vi "Tabellen.vi"(8 "Fehler (Eingang, kein Fehler)":errorcluster) -> (0 "Fehler (Ausgang)":errorcluster, 1 "Tabelle Kontroll Interferent":string[][](array[string]), 2 "Tabbelle Referenz Interferent":string[][](array[string]), 3 "Tabelle Komponente":string[][](array[string]), 4 "Istwerte Komponente":string[](array[string]), 5 "Fehler Komponente":string[](array[string]), 7 "Max. Fehler Komponente":dbl)   [LabVIEW 2020, in "EPA 1065.lvlib" / "HovaCAL Interference verificaton.lvlib"]
uses:
  HovaCAL Interference verificaton.lvlib
  Aktion Index uebersetzten.ctl
  Linearisierung V2/Aktion Lin Daten aufarbeiten.ctl
  Linearisierung V2/Linearisierung v2.lvlib
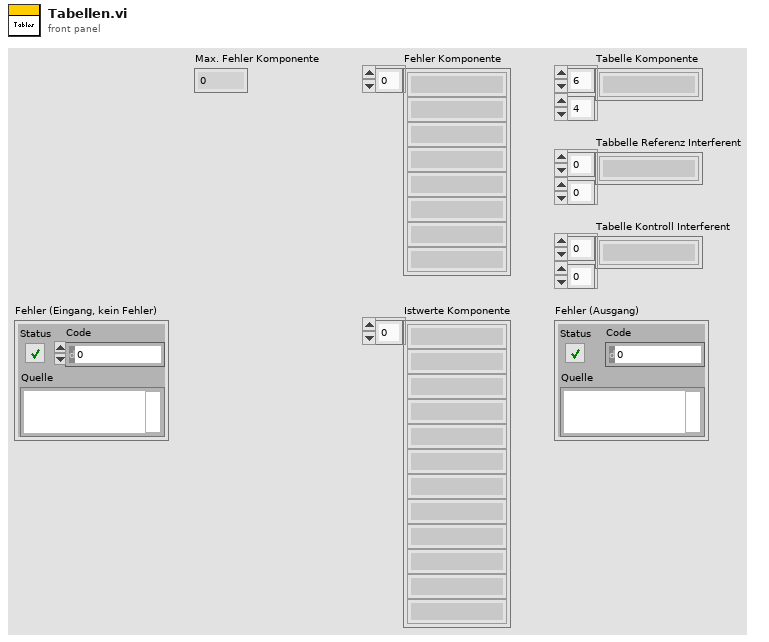
[diagram p1: front panel]
types:
  T1 = typedef "EPA 1065.lvlib/HovaCAL Interference verificaton.lvlib/Aktion Index uebersetzten.ctl" = enum16{"lesen", "schreiben", "auswerten", "Referenzwert", "KompIndex", "RefInterferIndex", "KontrInterfIndex"}
  T2 = typedef "Linearisierung v2.lvlib/Aktion Lin Daten aufarbeiten.ctl" = enum16{"lesen", "Protkolldaten", "speichern", "laden", "EPA auswerten", "Tabelle schreiben", "Lin auswerten", "Tab init", "Stufentabelle", "EPA aktiviert", "Nachbehandlung laden", "Tabelle löschen", "Istwerte löschen", "Zeile löschen", "Zeile einfügen", "LIN aktiviert", "LIN/EPA aktiv laden", "EGAK Tab", "LIN übernehmen", "Tab init ohne Stufen"}
  T3 = typedef "Linearisierung v2.lvlib/Eingabetabelle.ctl" = string[][]
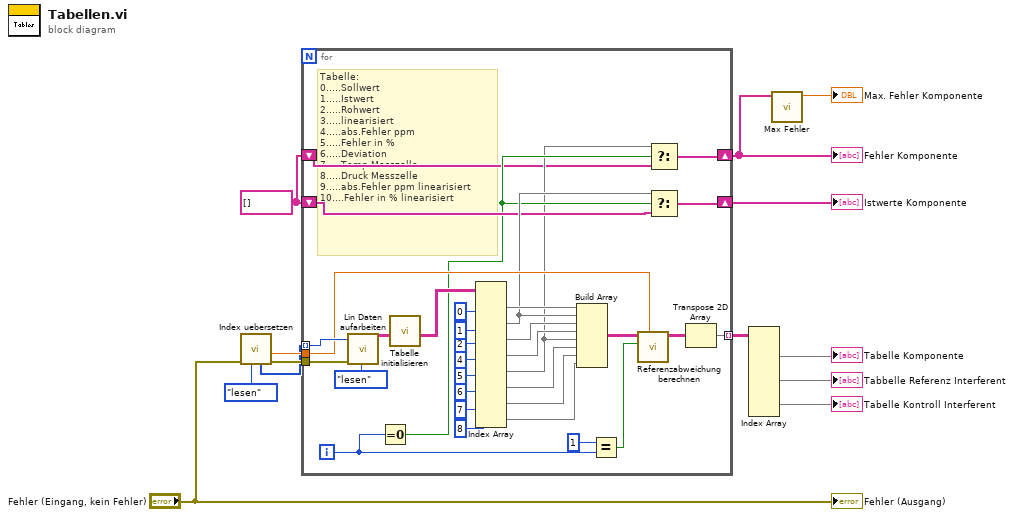
[diagram p0: block diagram]
diagram:
  w3 = string[] [] ("Tabelle")
  n1 = call "Index uebersetzen.vi"("Aktion"=Aktion_Index_uebersetzten."lesen", "error in (no error)"="Fehler (Eingang, kein Fehler)") -> ("error out"=w12:errorcluster, "Referenz out"=w7:sgl, "Komponenten Indices"=w5:i32[])  [unwired: 4 in, 3 out]
  n2 = for {
    tunnel: w12 -> [w45]
    tunnel: w5 -> [w44] mode=indexing
    tunnel: [w35] -> w11 mode=indexing
    tunnel: w7 -> [w23]
    shift-right: [w19] -> w4
    shift-left: w3 -> [w18]
    shift-right: [w15] -> w2
    shift-left: w3 -> [w14]
    i -> [w21]
    # "Tabelle:\n0.....Sollwert\n1.....Istwert\n2.....Rohwert\n3.....linearisiert\n4.....abs.Fehler ppm\n5.....Fehler in %\n6.....Deviation\n7.....Temp.Messzelle\n8.....Druck Messzelle\n9.....abs.Fehler ppm linearisiert\n10....Fehler in % linearisiert"
    n3 = call "Lin Daten aufarbeiten.vi"("Index (Seite)"=w44, "error in (no error)"=w45, "Aktionen"=Aktion_Lin_Daten_aufarbeiten."lesen") -> ("Eingabetabelle"=w43:T3)  [unwired: 14 in, 10 out]
    n4 = Equal To 0?(x=w21) -> (x = 0?=w17:bool)
    n5 = call "Tabelle initialisieren.vi"("Neue Tabelle"=w43) -> ("Tabelle"=w36:string[][])  [unwired: 10 in]
    n6 = Index Array(array=w36, index (col) #1=0 ("Deaktivierter Index (Spalte)"), index (col) #2=1 ("Index (Spalte)"), index (col) #3=2 ("Index (Spalte)"), index (col) #4=4 ("Index (Spalte)"), index (col) #5=5 ("Index (Spalte)"), index (col) #6=6 ("Index (Spalte)"), index (col) #7=7 ("Index (Spalte)"), index (col) #8=8 ("Index (Spalte)")) -> (element #1=w32:string[], element #2=w20:string[], element #3=w31:string[], element #4=w30:string[], element #5=w16:string[], element #6=w29:string[], element #7=w28:string[], element #8=w27:string[])  [unwired: 8 in]
    n7 = Build Array(w32, w20, w31, w30, w16, w29, w28, w27) -> (w25:string[][])
    n8 = Equal?(x=1, y=w21) -> (x = y?=w22:bool)
    n9 = call "Referenzabweichung berechnen.vi"("Referenz in"=w23, "Boolesch"=w22, "Array (Eingang)"=w25) -> ("Array (Ausgang)"=w24:string[][])  [unwired: 8 in]
    n10 = Select(t=w16, s=w17, f=w14) -> (s? t:f=w15:string[])
    n11 = Select(t=w20, s=w17, f=w18) -> (s? t:f=w19:string[])
    n12 = Transpose 2D Array(2D array=w24) -> (transposed array=w35:string[][])
  }
  "Istwerte Komponente" <- w4
  "Fehler Komponente" <- w2
  n13 = Index Array(array=w11) -> (element #1=→"Tabelle Komponente":string[][], element #2=→"Tabbelle Referenz Interferent":string[][], element #3=→"Tabelle Kontroll Interferent":string[][])  [unwired: 9 in]
  n14 = call "Max Fehler.vi"("Tabelle"=w2) -> ("max Fehler"=→"Max. Fehler Komponente":dbl)  [unwired: 10 in]
  "Fehler (Ausgang)" <- "Fehler (Eingang, kein Fehler)"
